vi "Read Currently Active Program.vi"(8 "ErrorIn":errorcluster, 11 "VISAIn":refnum<visa-resource-name>) -> (0 "ErrorOut":errorcluster, 2 "Data":string, 3 "VISAOut":refnum<visa-resource-name>)   [LabVIEW 2017, in "I28Drivers.lvlib"]
uses:
  I28Drivers.lvlib
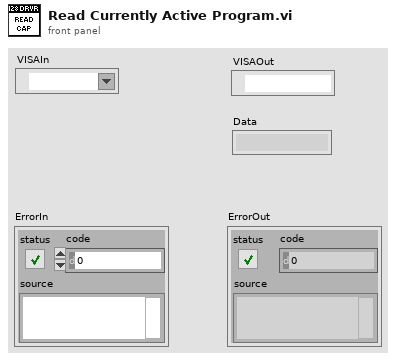
[diagram p1: front panel]
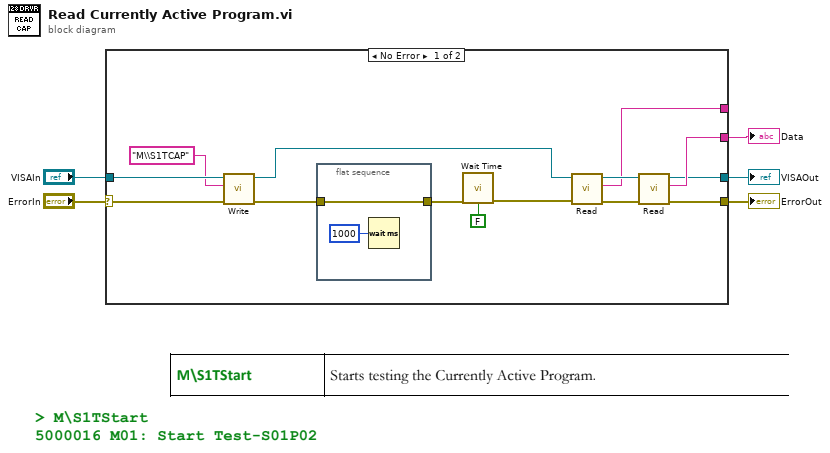
[diagram p0: block diagram]
diagram:
  n1 = case shown="No Error" "ErrorIn" {
    selector: "ErrorIn" -> [w19 w22]
    tunnel: "VISAIn" -> [w18 w23]
    tunnel: [w16 _] -> w3
    tunnel: [w15 w23] -> w1
    tunnel: [w14 w22] -> w2
    tunnel: [w11 _] -> _
    frame No Error {
      n2 = call "Write.vi"("ErrorIn"=w19, "Command"="M\\S1TCAP", "VISAIn"=w18) -> ("ErrorOut"=w7:errorcluster, "VISAOut"=w10:refnum<visa-resource-name>)  [unwired: 7 in]
      n3 = flat-sequence {
        tunnel: w7 -> [w21]
        tunnel: [w21] -> w6
        frame #0 {
          n4 = Wait (ms)(milliseconds to wait=u32 1000) -> ()  [unwired: 1 out]
        }
      }
      n5 = call "Wait Time.vi"("error in"=w6, "Set Time"=FALSE) -> ("error out"=w9:errorcluster)  [unwired: 13 in]
      n6 = call "Read.vi"("ErrorIn"=w9, "VISAIn"=w10) -> ("ErrorOut"=w13:errorcluster, "Data"=w11:string, "VISAOut"=w12:refnum<visa-resource-name>)  [unwired: 7 in]
      n7 = call "Read.vi"("ErrorIn"=w13, "VISAIn"=w12) -> ("ErrorOut"=w14:errorcluster, "Data"=w16:string, "VISAOut"=w15:refnum<visa-resource-name>)  [unwired: 7 in]
    }
    frame Error {
    }
  }
  "ErrorOut" <- w2
  "Data" <- w3
  "VISAOut" <- w1
